vi "Filter.vi"(8 "error in (no error)":errorcluster, 10 "Test Suite":refnum<class "LUnit Test Suite.lvclass">, 11 "Dashed Filter in":refnum<class "Dashed Filter.lvclass">) -> (0 "error out":errorcluster, 2 "Filtered Test Suite":refnum<class "LUnit Test Suite.lvclass">)   [LabVIEW 2020, in "Dashed Filter.lvclass"]
uses:
  Dashed Filter.lvclass
  API/LUnit Test Suite/LUnit Test Suite.lvclass
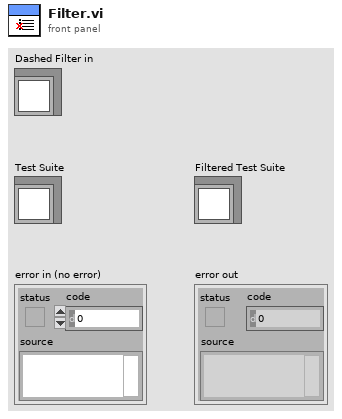
[diagram p1: front panel]
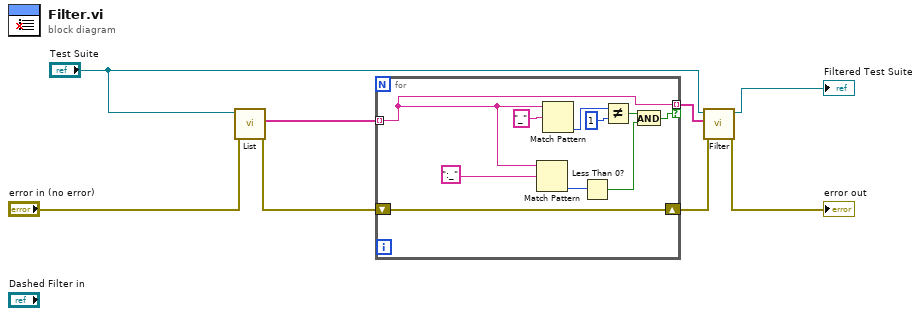
[diagram p0: block diagram]
diagram:
  n1 = call "List.vi"("error in (no error)"="error in (no error)", "LUnit Test Suite In"="Test Suite") -> ("error out"=w6:errorcluster, "List of Runnables"=w7:string[])  [unwired: 8 in]
  n2 = for {
    tunnel: w7 -> [w12] mode=indexing
    tunnel: [w12] -> w8 mode=indexing if=w10
    shift-right: [w18] -> w5
    shift-left: w6 -> [w18]
    n3 = Match Pattern(string=w12, regular expression=":_") -> (offset past match=w13:i32)  [unwired: 1 in, 3 out]
    n4 = Match Pattern(string=w12, regular expression="_") -> (offset past match=w16:i32)  [unwired: 1 in, 3 out]
    n5 = Less Than 0?(x=w13) -> (x < 0?=w9:bool)
    n6 = Not Equal?(x=w16, y=1) -> (x != y?=w14:bool)
    n7 = And(x=w14, y=w9) -> (x .and. y?=w10:bool)
  }
  n8 = call "Filter.vi"("error in (no error)"=w5, "Selected Runnables"=w8, "LUnit Test Suite In"="Test Suite") -> ("error out"=→"error out":errorcluster, "LUnit Test Suite Out"=→"Filtered Test Suite":refnum<class "LUnit Test Suite.lvclass">)  [unwired: 7 in]
